vi "Introspection Core.vi"(8 "error in (no error)":errorcluster, 11 "BNT_ULx-MCSV in":refnum<class "BNT_ULx-MCSV.lvclass">) -> (0 "error out":errorcluster, 1 "CSPPMessages":refnum<class "Message.lvclass">[](array[class]), 2 "Class History":string[](array[string]), 3 "BNT_ULx-MCSV out":refnum<class "BNT_ULx-MCSV.lvclass">)   [LabVIEW 2021, in "BNT_ULx.lvlib" / "BNT_ULx-MCSV.lvclass"]
doc: "This vi delivers a list with all messages this actor reacts to. \n\nNote that all inherited classes have to overwrite it."
uses:
  BNT_ULx-MCSV.lvclass
  <vilib>/ActorFramework/Message/Message.lvclass
  BNT_ULx-MCSV Messages/Readout Msg/Readout Msg.lvclass
  C:/Program Files (x86)/National Instruments/LabVIEW 2021/vi.lib/ActorFramework/Message/Message.lvclass
  BNT_ULx-MCSV Messages/Set Output Line Msg/Set Output Line Msg.lvclass
  BNT_ULx-MCSV Messages/Set Output Lines Msg/Set Output Lines Msg.lvclass
  BNT_ULx-MCSV Messages/Set Output Value Msg/Set Output Value Msg.lvclass
  BNT_ULx-MCSV Messages/Set Output Values Msg/Set Output Values Msg.lvclass
  CSPP_Core/Actors/CSPP_DeviceActor/CSPP_DeviceActor.lvclass
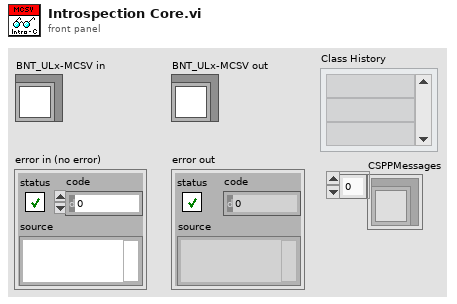
[diagram p1: front panel]
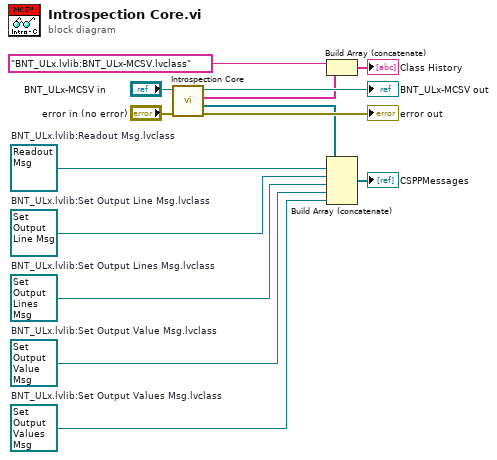
[diagram p0: block diagram]
diagram:
  w1 = refnum<class "Set Output Values Msg.lvclass"> refnum  # BNT_ULx.lvlib:Set Output Values Msg.lvclass
  w2 = refnum<class "Set Output Value Msg.lvclass"> refnum  # BNT_ULx.lvlib:Set Output Value Msg.lvclass
  w3 = refnum<class "Set Output Lines Msg.lvclass"> refnum  # BNT_ULx.lvlib:Set Output Lines Msg.lvclass
  w4 = refnum<class "Set Output Line Msg.lvclass"> refnum  # BNT_ULx.lvlib:Set Output Line Msg.lvclass
  w5 = refnum<class "Readout Msg.lvclass"> refnum  # BNT_ULx.lvlib:Readout Msg.lvclass
  n1 = call-parent "Introspection Core.vi"("Error In"="error in (no error)", "CSPP_DeviceActor in"="BNT_ULx-MCSV in") -> ("Error Out"=→"error out":errorcluster, "CSPP_Messages"=w9:refnum<class "Message.lvclass">[], "Class History"=w7:string[], "CSPP_DeviceActor out"=→"BNT_ULx-MCSV out":refnum<class "BNT_ULx-MCSV.lvclass">)  [unwired: 6 in]
  n2 = Build Array (concatenate)("BNT_ULx.lvlib:BNT_ULx-MCSV.lvclass", w7) -> (→"Class History":string[])
  n3 = Build Array (concatenate)(w9, w5, w4, w3, w2, w1) -> (→"CSPPMessages":refnum<class "Message.lvclass">[])
